vi "Close.vi"(8 "error in (no error)":errorcluster, 11 "uService Template in":refnum<class "TCP Server.lvclass">) -> (0 "error out":errorcluster, 3 "uService Template out":refnum<class "TCP Server.lvclass">)   [LabVIEW 2026, in "TALOS.lvlib" / "TCP Server.lvlib" / "TCP Server.lvclass"]
uses:
  TCP Server.lvclass
  TCP Server.lvclass/TCP Server.ctl
  Father of all uServices/Father of all uServices/Father of all uServices.lvclass
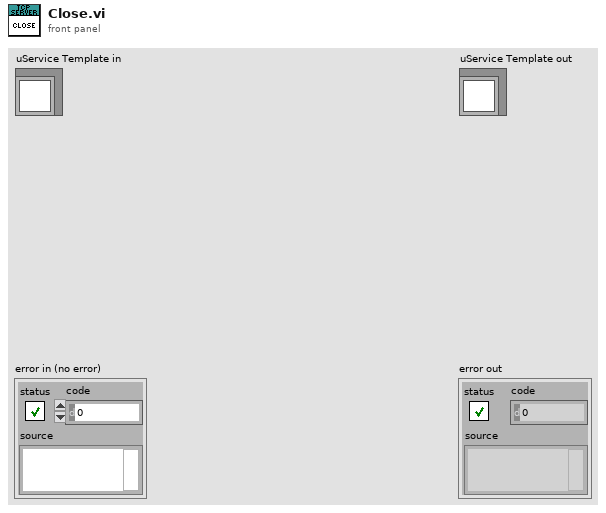
[diagram p1: front panel]
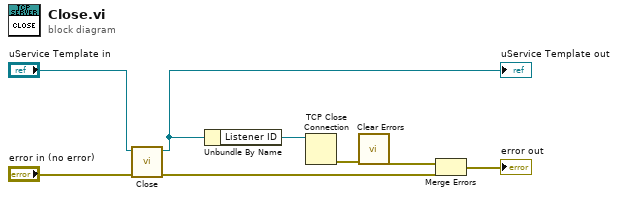
[diagram p0: block diagram]
diagram:
  n1 = call-parent "Close.vi"("error in (no error)"="error in (no error)", "uService Template in"="uService Template in") -> ("error out"=w3:errorcluster, "uService Template out"=w6:refnum<class "TCP Server.lvclass">)  [unwired: 8 in]
  "uService Template out" <- w6
  n2 = Unbundle By Name(w6) -> ("Listener ID"=w5:refnum<k5>)
  n3 = TCP Close Connection(connection ID=w5) -> (error out=w4:errorcluster)  [unwired: 2 in, 1 out]
  n4 = call <vilib>:"Clear Errors.vi"("error in (no error)"=w4) -> ("error out"=w2:errorcluster)  [unwired: 5 in, 1 out]
  n5 = Merge Errors(w2, w3) -> (→"error out":errorcluster)
